vi "Get Window HWnd.vi"(8 "error in (no error)":errorcluster, 11 "Window Name":string) -> (0 "error out":errorcluster, 3 "HWnd Out":u32)   [LabVIEW 2011]
doc: "This VI will use the FindWindow API function to retrieve a window refnum for the window identified by window name. 'window name' is the text appearing in the title bar of a window. If the window cannot be found, the window refnum out will be 'Not a Window Refnum', and an error will occur."
uses:
  User32.dll
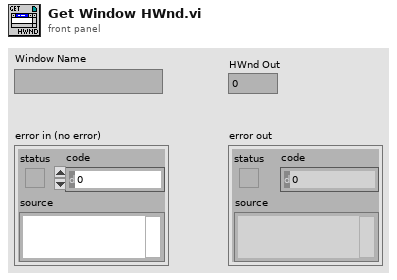
[diagram p1: front panel]
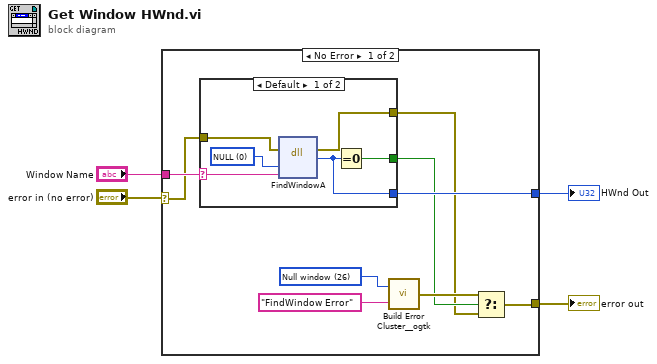
[diagram p0: block diagram]
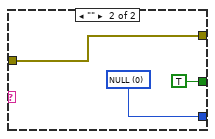
[diagram p2: hidden frame]
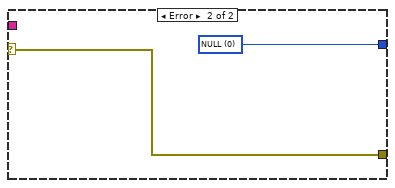
[diagram p3: hidden frame]
diagram:
  n1 = case shown="No Error" "error in (no error)" {
    selector: "error in (no error)" -> [w11 w23]
    tunnel: [w5 w23] -> w1
    tunnel: [w13 w24] -> w2
    tunnel: "Window Name" -> [w12 _]
    frame No Error {
      w8 = 26 items=["No error", "Argument error", "Memory is full", "Out of zone", "End of file", "File already open", "Generic file I/O error", "File not found", "File permission error", "Disk is full", "Duplicate path", "Too many files open", "System feature not enabled", "Resource file not found", "Cannot add resource", "Resource not found", "Image not found", "Image memory error", "Pen does not exist", "Config type invalid", "Config token not found", "Config parse error", "Config memory error", "Bad external code format", "Bad external code offset", "External code not present", "Null window", "Destroy window error", "Null menu", "Print aborted", "Bad print record", "Print driver error", "Windows error during printing", "Memory error during printing", "Print dialog error", "Generic print error", "Invalid device refnum", "Device not found", "Device parameter error", "Device unit error", "Cannot open device", "Device call aborted", "Generic error", "Cancelled by user", "Object ID too low", "Object ID too high", "Object not in heap", "Unknown heap", "Unknown object (invalid DefProc)", "Unknown object (DefProc not in table)", "Message out of range", "Invalid (null) method", "Unknown message", "Manager call not supported", "Bad address", "Network operation in progress", "Network operation timed out", "Connection is busy", "Network attribute not supported", "Network error", "Address in use", "System out of memory", "Connection aborted", "Connection refused", "Not connected", "Already connected", "Connection closed", "Initialization error (interapplication manager)", "Bad occurrence", "Wait on unbound occurrence handler", "Occurrence queue overflow", "Datalog type conflict", "Unused", "Unrecognized type (interapplication manager)", "Memory corrupt", "Failed to make temporary DLL", "Old CIN version", "Drag socket not found", "Failed to load drop-object", "Failed to register OLE object", "Failed to release OLE object", "Format specifier type mismatch", "Unknown format specifier", "Too few format specifiers", "Too many format specifiers", "Scan failed", "Newer CIN version", "Error converting to variant", "Runtime menu error", "Password tampered", "Variant attribute not found", "Incompatible variant data type", "Event data is not available", "Event Store is not present", "Occurrence is not found", "Event Queue is not created", "Event info is not available", "Refnum passed is NULL", "Error retrieving Class GUID", "Error retrieving CoClass GUID", "Error retrieving TypeLib GUID.", "Bad built application magic bytes.", "Specific driver is different from the specific driver associated with the Logical Name.", "There is no session opened to the class driver.", "Max Error", "MAX - Error with config objects", "MAX - Error loading configuration", "MAX - Group not supported"]
      n2 = case shown="Default" w12 {
        selector: w12 -> [w16 _]
        tunnel: [w19 w22] -> w13
        tunnel: [w18 TRUE] -> w7
        tunnel: w11 -> [w15 w20]
        tunnel: [w14 w20] -> w6
        frame Default {
          w17 = 0 items=["NULL"]
          n3 = dll-call lib="user32.dll" fn="FindWindowA" label="FindWindow"(error in=w15, "lpszClassName"=w17, "lpszWindowName"=w16) -> (error out=w14:errorcluster, "hWnd"=w19:u32)  [unwired: 4 in, 1 out]
          n4 = Equal To 0?(x=w19) -> (x = 0?=w18:bool)
        }
        frame "" {
          w22 = u32 0 items=["NULL"]
        }
      }
      n5 = call <userlib>:"Build Error Cluster__ogtk.vi"("String to Prepend to source (\"\")"="FindWindow Error" ("String to Prepend to source (\"\")"), "code"=w8) -> ("error out"=w9:errorcluster)
      n6 = Select(t=w9, s=w7, f=w6) -> (s? t:f=w5:errorcluster)
    }
    frame Error {
      w24 = u16 0 items=["NULL"]
    }
  }
  "HWnd Out" <- w2
  "error out" <- w1
